vi "Create_local_data_subdirectory.vi"(7 "Suffix data path":string, 8 "error in (no error)":errorcluster, 11 "Local file path":path=path "C:/Users/ZODI/Documents/LabVIEW Data/FITS Files") -> (0 "error out":errorcluster, 2 "Local file full path updated":path, 3 "Created (existed before) data path)":path, 5 "file or folder exists?":bool)   [LabVIEW 2022 SP3]
panel:
  out "suffix length":i32
  out "Created successfully":bool
  out "before substring":string
  out "after substring":string
  out "FITS file name":string
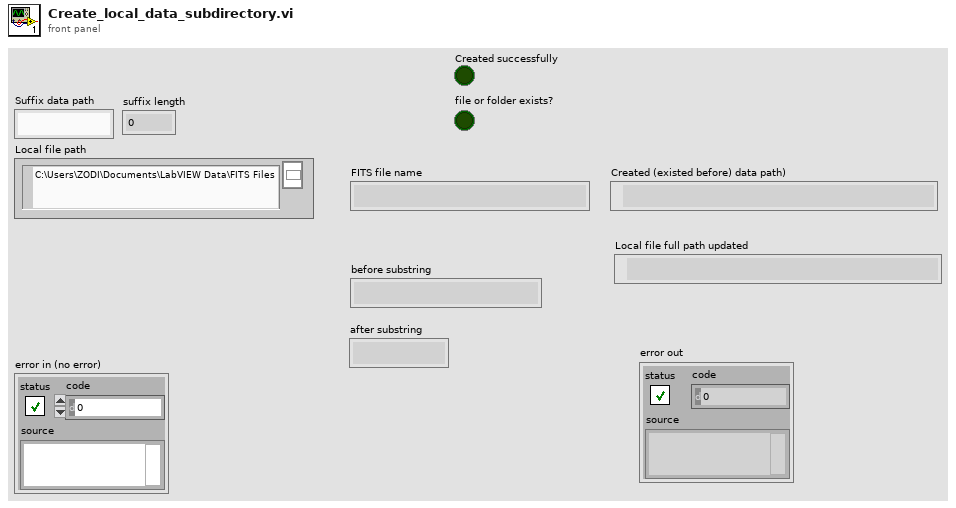
[diagram p1: front panel]
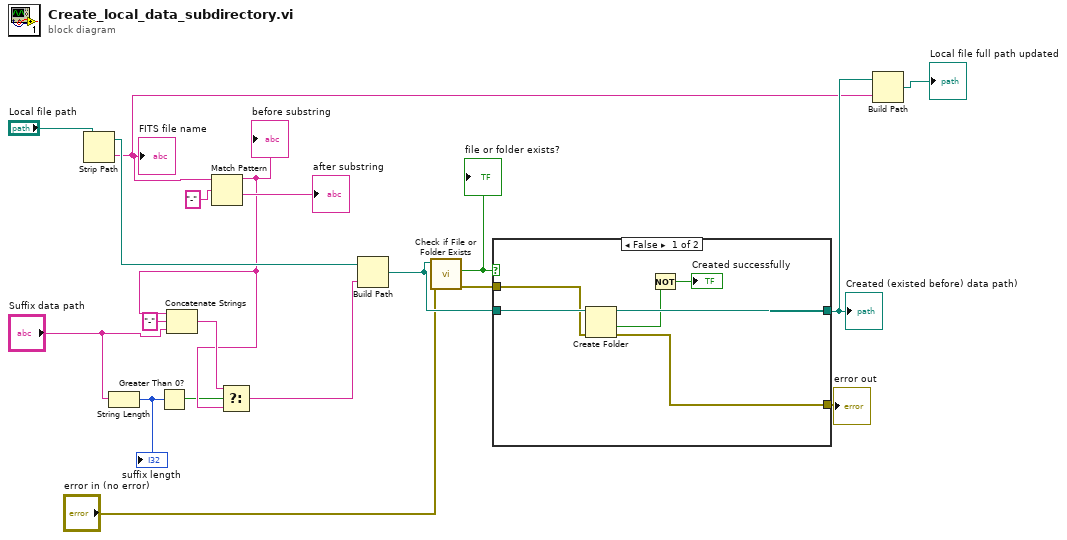
[diagram p0: block diagram]
diagram:
  n1 = Strip Path(path="Local file path") -> (stripped path=w14:path, name=w1:string)
  "FITS file name" <- w1
  n2 = String Length(string="Suffix data path") -> (length=w12:i32)
  "suffix length" <- w12
  n3 = Greater Than 0?(x=w12) -> (x > 0?=w7:bool)
  n4 = Match Pattern(string=w1, regular expression="-" ("search string")) -> (before substring=w8:string, after substring=→"after substring":string)  [unwired: 1 in, 2 out]
  "before substring" <- w8
  n5 = Concatenate Strings(w8, "-" ("string"), "Suffix data path") -> (w9:string)
  n6 = Select(t=w9, s=w7, f=w8) -> (s? t:f=w6:string)
  n7 = Build Path(base path=w14, name or relative path=w6) -> (appended path=w15:path)
  n8 = call <vilib>:"Check if File or Folder Exists.vi"("error in (no error)"="error in (no error)", "path"=w15) -> ("error out"=w5:errorcluster, "file or folder exists?"=w16:bool)  [unwired: 7 in, 1 out]
  "file or folder exists?" <- w16
  n9 = case shown="False" w16 {
    tunnel: w15 -> [w25 w27]
    tunnel: [w24 w27] -> w2
    tunnel: w5 -> [w23 w26]
    tunnel: [w22 w26] -> w4
    frame False {
      n10 = Create Folder(path (use dialog)=w25, error in=w23) -> (created path=w24:path, cancelled=w21:bool, error out=w22:errorcluster)  [unwired: 1 in]
      n11 = Not(x=w21) -> (.not. x?=→"Created successfully":bool)
    }
    frame True {
    }
  }
  "Created (existed before) data path)" <- w2
  "error out" <- w4
  n12 = Build Path(base path=w2, name or relative path=w1) -> (appended path=→"Local file full path updated":path)
